vi "Post_Measure_Analysis.vi"(0 "VISA Refnum in":refnum<visa-resource-name>, 1 "Var2 step settings":T2, 2 "Sample Properties:":T4, 3 "Vname":string, 4 "Execute?":bool, 5 "Header Strings":T3, 6 "Var1 sweep settings":T1, 7 "error in (no error)":errorcluster, 8 "Id Vg Data":cluster{"trace":dbl[], "trace":dbl[]}, 9 "Dielectric Constant":dbl, 10 "Gate Current":cluster{"trace":dbl[], "trace":dbl[]}[](array[cluster]), 11 "NumPts":dbl, 12 "Input Path":path, 13 "Ambient Temp (Y/N)":bool=TRUE, 14 "Graph Cluster in":T5) -> (16 "File out":path, 18 "Vg Data":dbl[](array[numeric]), 20 "Header out":string, 21 "Vd Data":dbl[](array[numeric]), 22 "Id Data":dbl[](array[numeric]), 23 "Graph Cluster out":T5, 24 "Device Properties Out":T6, 25 "Check Cluster":T7, 27 "error out":errorcluster)   [LabVIEW 2012]
uses:
  <vilib>/Utility/file.llb/Write To Spreadsheet File (DBL).vi
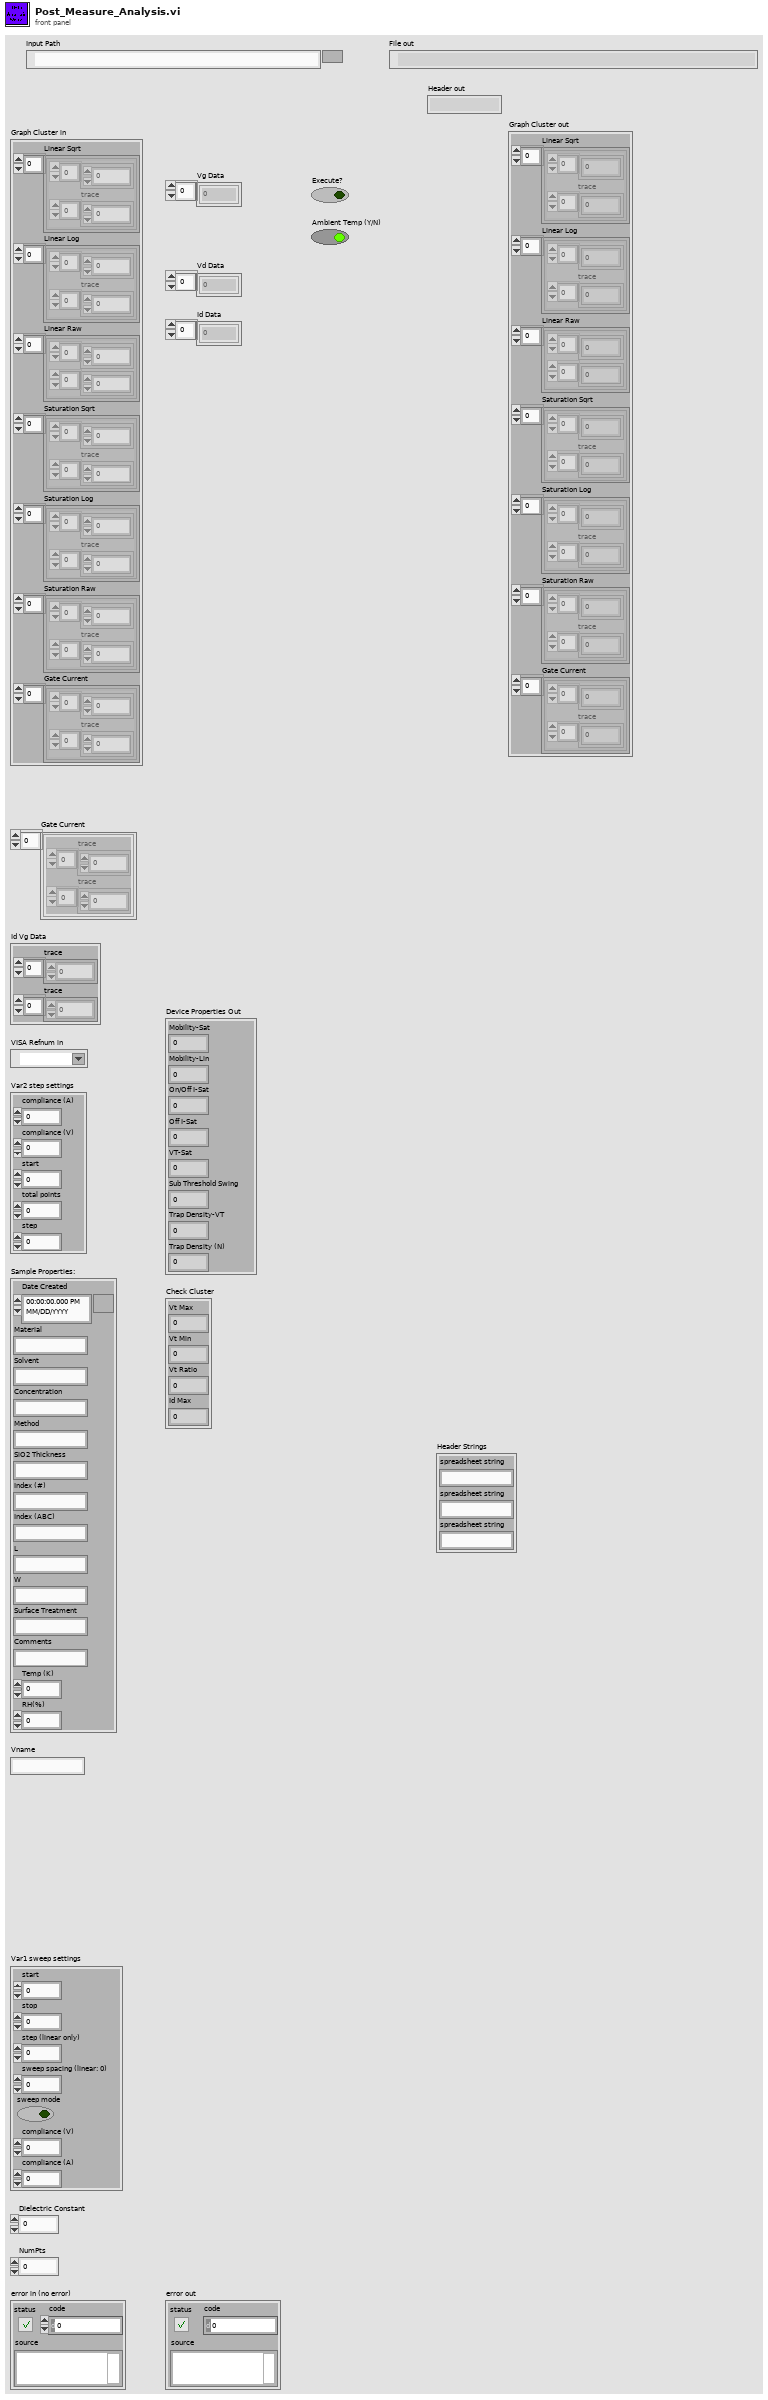
[diagram p1: front panel]
types:
  T1 = cluster{"start":dbl, "stop":dbl, "step (linear only)":dbl, "sweep spacing (linear: 0)":u16, "sweep mode":bool, "compliance (V)":dbl, "compliance (A)":dbl}
  T2 = cluster{"compliance (A)":dbl, "compliance (V)":dbl, "start":dbl, "total points":u16, "step":dbl}
  T3 = cluster{"spreadsheet string":string, "spreadsheet string":string, "spreadsheet string":string}
  T4 = cluster{"Date Created":timestamp, "Material":string, "Solvent":string, "Concentration":string, "Method":string, "SiO2 Thickness":string, "Index (#)":string, "Index (ABC)":string, "L":string, "W":string, "Surface Treatment":string, "Comments":string, "Temp (K)":dbl, "RH(%)":dbl}
  T5 = cluster{"Linear Sqrt":cluster{dbl[], "trace":dbl[]}[], "Linear Log":cluster{dbl[], "trace":dbl[]}[], "Linear Raw":cluster{dbl[], dbl[]}[], "Saturation Sqrt":cluster{dbl[], "trace":dbl[]}[], "Saturation Log":cluster{dbl[], "trace":dbl[]}[], "Saturation Raw":cluster{dbl[], "trace":dbl[]}[], "Gate Current":cluster{dbl[], "trace":dbl[]}[]}
  T6 = cluster{"Mobility-Sat":dbl, "Mobility-Lin":dbl, "On/Off I-Sat":dbl, "Off I-Sat":dbl, "VT-Sat":dbl, "Sub Threshold Swing":dbl, "Trap Density-VT":dbl, "Trap Density (N)":dbl}
  T7 = cluster{"Vt Max":dbl, "Vt Min":dbl, "Vt Ratio":dbl, "Id Max":dbl}
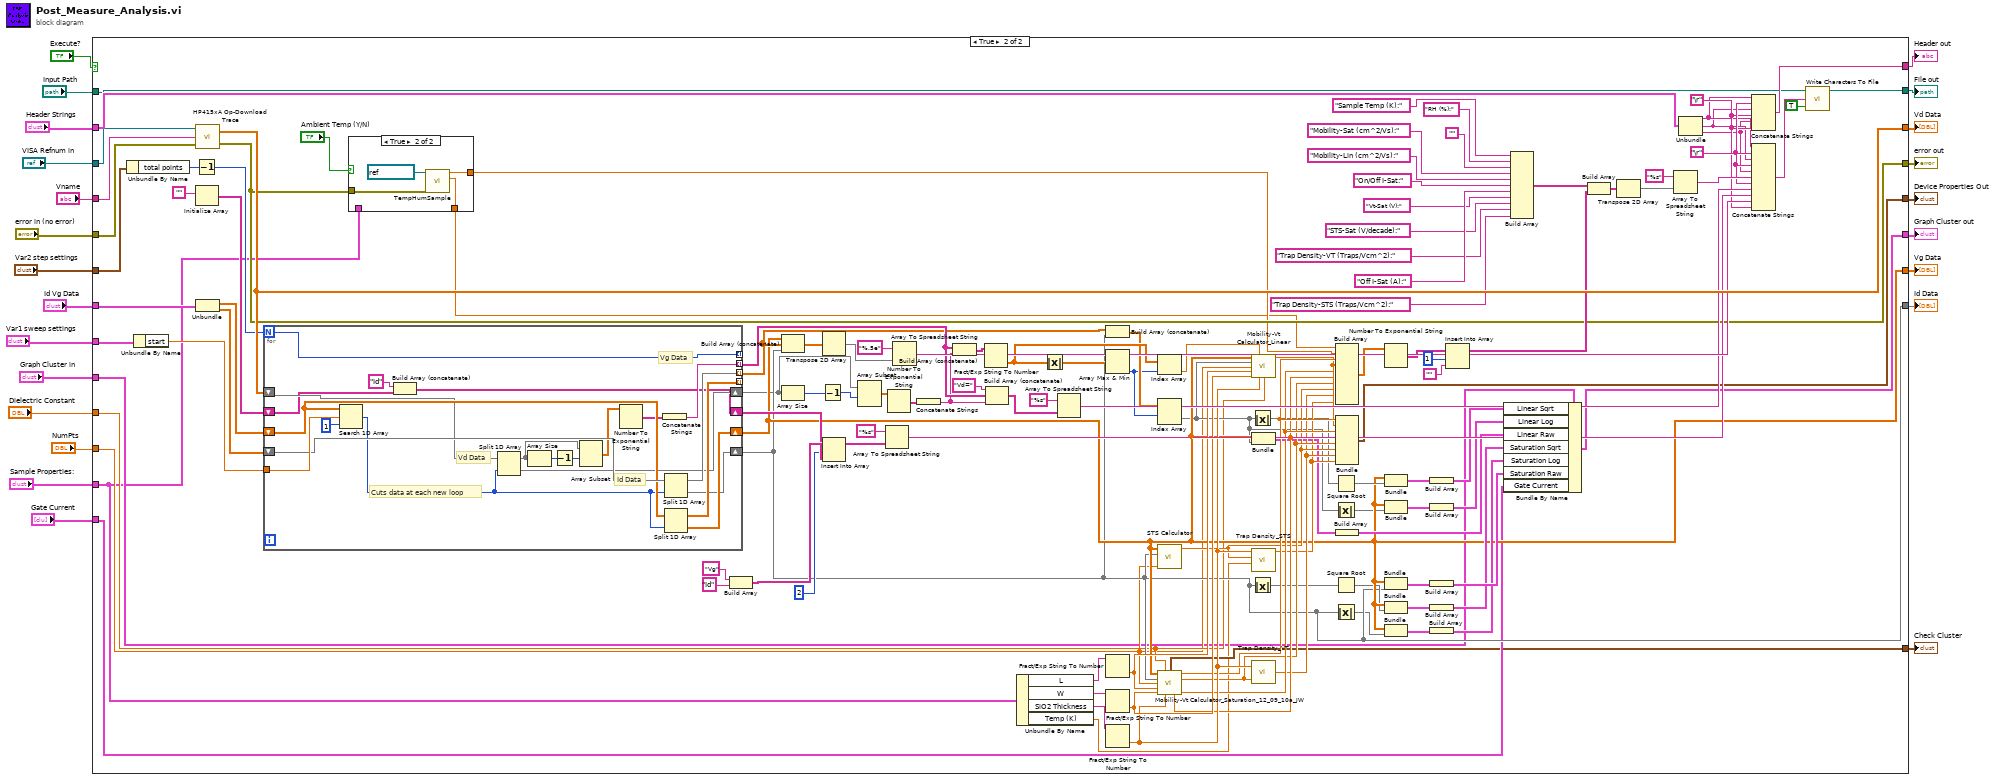
[diagram p0: block diagram]
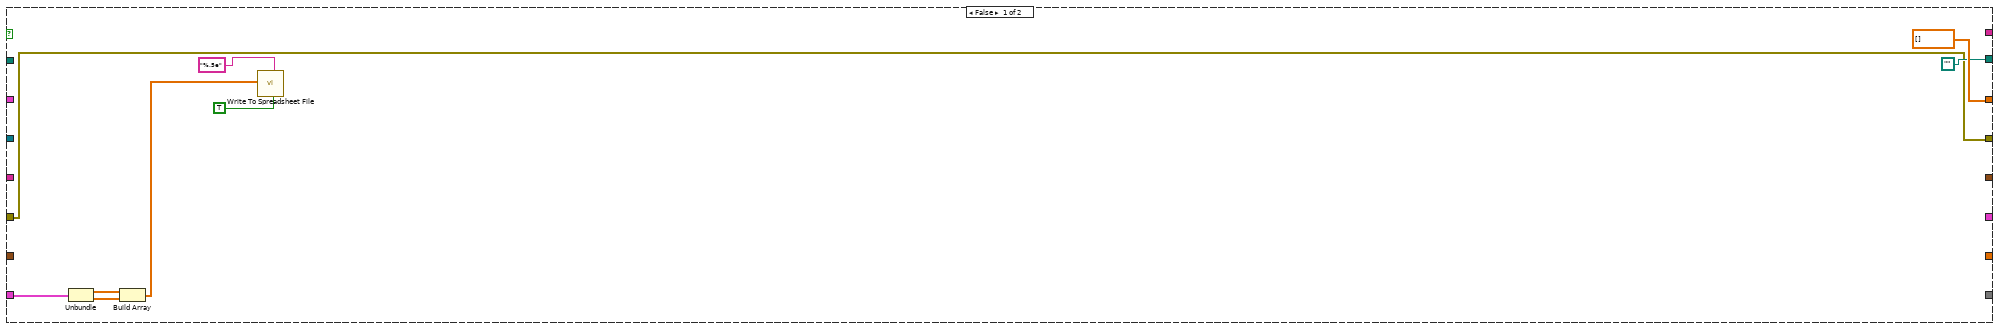
[diagram p2: hidden frame]
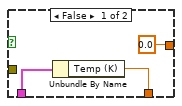
[diagram p3: hidden frame]
diagram:
  n1 = case shown="True" "Execute?" {
    tunnel: "VISA Refnum in" -> [_ w35]
    tunnel: "error in (no error)" -> [w24 w153]
    tunnel: [w24 w63] -> w1
    tunnel: "Vname" -> [_ w36]
    tunnel: [dbl[] [] ("trace") w152] -> w2
    tunnel: [_ w78] -> w4
    tunnel: [_ w73] -> w5
    tunnel: "Gate Current" -> [_ w70]
    tunnel: [_ w65] -> w8
    tunnel: "Var1 sweep settings" -> [_ w60]
    tunnel: "Var2 step settings" -> [_ w58]
    tunnel: "Header Strings" -> [_ w55]
    tunnel: "Sample Properties:" -> [_ w34]
    tunnel: "Id Vg Data" -> [w28 w48]
    tunnel: [_ w45] -> w16
    tunnel: [_ w44] -> w17
    tunnel: [_ w43] -> w18
    tunnel: "Dielectric Constant" -> [_ w42]
    tunnel: "NumPts" -> [_ w40]
    tunnel: [path "" w39] -> w21
    tunnel: "Input Path" -> [_ w38]
    tunnel: "Graph Cluster in" -> [_ w37]
    frame False {
      n2 = Unbundle(w28) -> ("trace"=w27:dbl[], "trace"=w26:dbl[])
      n3 = Build Array(w27, w26) -> (w30:dbl[][])
      n4 = call-poly <vilib>:"Write To Spreadsheet File.vi"("transpose? (no:F)"=TRUE ("append to file? (new file:F)"), "format (%.3f)"="%.5e", "2D data"=w30) -> ()  [unwired: 5 in, 1 out]
    }
    frame True {
      w68 = "\r"
      w69 = "\r"
      n5 = Unbundle By Name(w58) -> ("total points"=w57:u16)
      n6 = Unbundle By Name(w60) -> ("start"=w59:dbl)
      n7 = Decrement(x=w57) -> (x-1=w56:u16)
      n8 = Initialize Array("") -> (w133:string[])  [unwired: 1 in]
      n9 = call "HP415xA Op-Download Trace.vi"("error in (no error)"=w153, "trace (variable) name"=w36, "VISA session"=w35) -> ("error out"=w63:errorcluster, "trace"=w152:dbl[])
      n10 = Unbundle(w48) -> ("trace"=w47:dbl[], "trace"=w46:dbl[])
      n11 = for {
        N: w56 -> [w164]
        shift-right: [w181] -> w78
        shift-left: w47 -> [w177]
        tunnel: w59 -> [w183]
        tunnel: [w182] -> _ mode=indexing
        shift-right: [w178] -> w73
        shift-left: w46 -> [w180]
        tunnel: [w179] -> w115 mode=indexing
        shift-right: [w174] -> w67
        shift-left: w152 -> [w176]
        tunnel: [w168] -> w116 mode=indexing
        shift-right: [w167] -> w137
        shift-left: w133 -> [w166]
        tunnel: [w164] -> _ mode=indexing
        # "Cuts data at each new loop"
        # "Id Data"
        # "Vd Data"
        # "Vg Data"
        n12 = Search 1D Array(1D array=w177, element=w183, start index (0)=1) -> (index of element=w175:i32)
        n13 = Build Array (concatenate)("Id", w166) -> (w167:string[])
        n14 = Split 1D Array(array=w176, index=w175) -> (first subarray=w172:dbl[], second subarray=w174:dbl[])
        n15 = Array Size(array=w172) -> (size(s)=w171:i32)
        n16 = Decrement(x=w171) -> (x-1=w170:i32)
        n17 = Array Subset(array=w172, index=w170) -> (w173:dbl[])  [unwired: 1 in]
        n18 = Number To Exponential String(number=w173) -> (E-format string=w169:string[])  [unwired: 3 in]
        n19 = Concatenate Strings(w169) -> (w168:string)
        n20 = Split 1D Array(array=w180, index=w175) -> (first subarray=w179:dbl[], second subarray=w178:dbl[])
        n21 = Split 1D Array(array=w177, index=w175) -> (first subarray=w182:dbl[], second subarray=w181:dbl[])
      }
      n22 = case shown="True" "Ambient Temp (Y/N)" {
        tunnel: w63 -> [_ w163]
        tunnel: [0.0 w161] -> w62
        tunnel: [w158 w160] -> w61
        tunnel: w34 -> [w157 _]
        frame False {
          n23 = Unbundle By Name(w157) -> ("Temp (K)"=w158:dbl)
        }
        frame True {
          n24 = call "TempHumSample.vi"("VISA resource name"=refnum<visa-resource-name> "COM4", "error in (no error)"=w163) -> ("CurHum"=w161:dbl, "CurTemp"=w160:dbl)  [unwired: 6 in, 1 out]
        }
      }
      n25 = Build Array("Vg", "Id") -> (w138:string[])
      n26 = Build Array (concatenate)(w78, w115, w73) -> (w156:dbl[][])
      n27 = Array Size(array=w67) -> (size(s)=w147:i32)
      n28 = Decrement(x=w147) -> (x-1=w146:i32)
      n29 = Transpose 2D Array(2D array=w156) -> (transposed array=w154:dbl[][])
      n30 = Insert Into Array(array=w138, index=2, new element=w137) -> (w136:string[])
      n31 = Array Subset(array=w67, index=w146) -> (w145:dbl[])  [unwired: 1 in]
      n32 = Array To Spreadsheet String(array=w136, 3:"%s") -> (spreadsheet string=w142:string)  [unwired: 1 in]
      n33 = Number To Exponential String(number=w145) -> (E-format string=w141:string[])  [unwired: 3 in]
      n34 = Array To Spreadsheet String(array=w154, 3:"%.5e" ("format string")) -> (spreadsheet string=w149:string)  [unwired: 1 in]
      n35 = Concatenate Strings(w141) -> (w66:string)
      n36 = Build Array (concatenate)(w116, w66) -> (w114:string[])
      n37 = Fract/Exp String To Number(string=w114) -> (number=w103:dbl[])  [unwired: 3 in, 1 out]
      n38 = Build Array (concatenate)("Vd=", w116, w66) -> (w144:string[])
      n39 = Unbundle By Name(w34) -> ("L"=w50:string, "W"=w49:string, "SiO2 Thickness"=w51:string, "Temp (K)"=w41:dbl)
      n40 = Absolute Value(x=w103) -> (abs(x)=w104:dbl[])
      n41 = Array To Spreadsheet String(array=w144, 3:"%s") -> (spreadsheet string=w148:string)  [unwired: 1 in]
      n42 = Build Array (concatenate)(w115, w73) -> (w101:dbl[][])
      n43 = Array Max & Min(array=w104) -> (min index (indices)=w100:i32)  [unwired: 3 out]
      n44 = Fract/Exp String To Number(string=w50) -> (number=w118:dbl)  [unwired: 3 in, 1 out]
      n45 = Fract/Exp String To Number(string=w49) -> (number=w119:dbl)  [unwired: 3 in, 1 out]
      n46 = Fract/Exp String To Number(string=w51) -> (number=w113:dbl)  [unwired: 3 in, 1 out]
      n47 = Index Array(array=w103, index=w100) -> (element=w102:dbl)
      n48 = Index Array(array=w101, index (row)=w100) -> (element=w75:dbl[])  [unwired: 1 in]
      n49 = call "STS Calculator.vi"("NumPts"=w40, "Saturation Id"=w73, "Vg Column"=w78) -> ("Sub Threshold Swing"=w107:dbl)  [unwired: 5 in, 3 out]
      n50 = call "Mobility-Vt Calculator_Saturation_12_09_10a_JW.vi"("Vg Column"=w78, "Dielectric Constant"=w42, "Sat Id Column"=w73, "NumPts"=w40, "Length"=w118, "Width"=w119, "Dielectric Thickness"=w113) -> ("Check Cluster"=w43:T7, "Mobility-Sat"=w112:dbl, "VT-Sat"=w108:dbl, "Off I-Sat"=w109:dbl, "On/Off I-Sat"=w110:dbl)  [unwired: 4 out]
      n51 = Absolute Value(x=w75) -> (abs(x)=w80:dbl[])
      n52 = Absolute Value(x=w73) -> (abs(x)=w77:dbl[])
      n53 = call "Mobility-Vt Calculator_Linear.vi"("Vg Column"=w78, "Vd"=w102, "Lin Id Column"=w75, "NumPts"=w40, "Length"=w118, "Width"=w119, "Dielectric Thickness"=w113, "Dielectric Constant"=w42) -> ("Mobility-Lin"=w111:dbl)  [unwired: 1 in, 6 out]
      n54 = Bundle("trace"=w78, w75) -> (w89:cluster{"trace":dbl[], dbl[]})  [unwired: 1 in]
      n55 = call "Trap Density_STS.vi"("Temp (T) [K]"=w41, "S.T.S. (S)"=w107, "Dielectric"=w113) -> ("Trap Density (N)"=w105:dbl)  [unwired: 8 in]
      n56 = call "Trap Density_VT.vi"("VT"=w108, "Dielectric"=w113) -> ("Trap Density-VT"=w106:dbl)
      n57 = Square Root(x=w80) -> (sqrt(x)=w79:dbl[])
      n58 = Absolute Value(x=w75) -> (abs(x)=w74:dbl[])
      n59 = Square Root(x=w77) -> (sqrt(x)=w76:dbl[])
      n60 = Absolute Value(x=w73) -> (abs(x)=w72:dbl[])
      n61 = Build Array(w61, w62, w112, w111, w110, w109, w108, w107, w106, w105) -> (w130:dbl[])
      n62 = Bundle("Mobility-Sat"=w112, "Mobility-Lin"=w111, "On/Off I-Sat"=w110, "Off I-Sat"=w109, "VT-Sat"=w108, "Sub Threshold Swing"=w107, "Trap Density-VT"=w106, "Trap Density (N)"=w105) -> (w44:T6)  [unwired: 1 in]
      n63 = Build Array(w89) -> (w88:cluster{"trace":dbl[], dbl[]}[])
      n64 = Number To Exponential String(number=w130) -> (E-format string=w98:string[])  [unwired: 3 in]
      n65 = Bundle("trace"=w78, w79) -> (w82:cluster{"trace":dbl[], dbl[]})  [unwired: 1 in]
      n66 = Bundle("trace"=w78, w74) -> (w83:cluster{"trace":dbl[], dbl[]})  [unwired: 1 in]
      n67 = Bundle("trace"=w78, "trace"=w73) -> (w91:cluster{"trace":dbl[], "trace":dbl[]})  [unwired: 1 in]
      n68 = Bundle("trace"=w78, w76) -> (w87:cluster{"trace":dbl[], dbl[]})  [unwired: 1 in]
      n69 = Bundle("trace"=w78, w72) -> (w86:cluster{"trace":dbl[], dbl[]})  [unwired: 1 in]
      n70 = Build Array(w82) -> (w81:cluster{"trace":dbl[], dbl[]}[])
      n71 = Build Array(w83) -> (w71:cluster{"trace":dbl[], dbl[]}[])
      n72 = Build Array(w91) -> (w90:cluster{"trace":dbl[], "trace":dbl[]}[])
      n73 = Build Array(w87) -> (w84:cluster{"trace":dbl[], dbl[]}[])
      n74 = Build Array(w86) -> (w85:cluster{"trace":dbl[], dbl[]}[])
      n75 = Insert Into Array(array=w98, index=1, new element="") -> (w95:string[])
      n76 = Bundle By Name(cluster=w37, "Linear Sqrt"=w81, "Linear Log"=w71, "Linear Raw"=w88, "Saturation Sqrt"=w84, "Saturation Log"=w85, "Saturation Raw"=w90, "Gate Current"=w70) -> (w45:T5)
      n77 = Build Array("Sample Temp (K):", "RH (%):", "", "Mobility-Sat (cm^2/Vs):", "Mobility-Lin (cm^2/Vs):", "On/Off I-Sat:", "Off I-Sat (A):", "Vt-Sat (V):", "STS-Sat (V/decade):", "Trap Density-VT (Traps/Vcm^2):", "Trap Density-STS (Traps/Vcm^2):") -> (w131:string[])
      n78 = Build Array(w131, w95) -> (w94:string[][])
      n79 = Transpose 2D Array(2D array=w94) -> (transposed array=w93:string[][])
      n80 = Array To Spreadsheet String(array=w93, 3:"%s") -> (spreadsheet string=w128:string)  [unwired: 1 in]
      n81 = Unbundle(w55) -> ("spreadsheet string"=w54:string, "spreadsheet string"=w53:string, "spreadsheet string"=w52:string)
      n82 = Concatenate Strings(w54, w69, w53, w68, w52, w68) -> (w65:string)
      n83 = Concatenate Strings(w54, w69, w53, w69, w52, w128, w69, w148, w142, w149, w68) -> (w151:string)
      n84 = call <vilib>:"Write Characters To File.vi"("append to file? (new file:F)"=TRUE, "character string"=w151, "file path (dialog if empty)"=w38) -> ("new file path (Not A Path if cancelled)"=w39:path)  [unwired: 2 in]
    }
  }
  "File out" <- w21
  "Check Cluster" <- w18
  "Device Properties Out" <- w17
  "Graph Cluster out" <- w16
  "Header out" <- w8
  "Id Data" <- w5
  "Vg Data" <- w4
  "Vd Data" <- w2
  "error out" <- w1
